vi "Get Sender.vi"(11 "Go To Destroy Msg in":refnum<class "Go To Destroy Msg.lvclass">) -> (2 "Sender":refnum<class "Sender.lvclass">)   [LabVIEW 2020, in "jettl.lvlib" / "Go To Destroy Msg.lvlib" / "Go To Destroy Msg.lvclass"]
uses:
  Go To Destroy Msg.lvclass
  Sender/Sender/Sender.lvclass
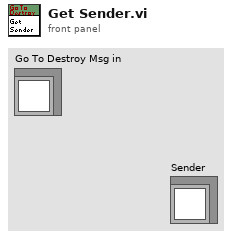
[diagram p1: front panel]
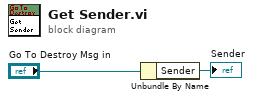
[diagram p0: block diagram]
diagram:
  n1 = Unbundle By Name("Go To Destroy Msg in") -> ("Sender"=→"Sender":refnum<class "Sender.lvclass">)
